vi "Mem_MemoryToLvData_NOPTR.vi"(7 "Type":variant, 8 "error in (no error)":errorcluster, 10 "ByteArray":u8[](array[numeric])) -> (0 "error out":errorcluster, 1 "Supported Type?":bool, 2 "data":variant, 4 "ByteArray Left":u8[](array[numeric]))   [LabVIEW 2019, in "Memory Data Access.lvlib"]
uses:
  Memory Data Access.lvlib
  <vilib>/Utility/Data Type/Type Definitions/Data Type.ctl
  Global/Global.vi
  <vilib>/Utility/Data Type/NI_Data Type.lvlib
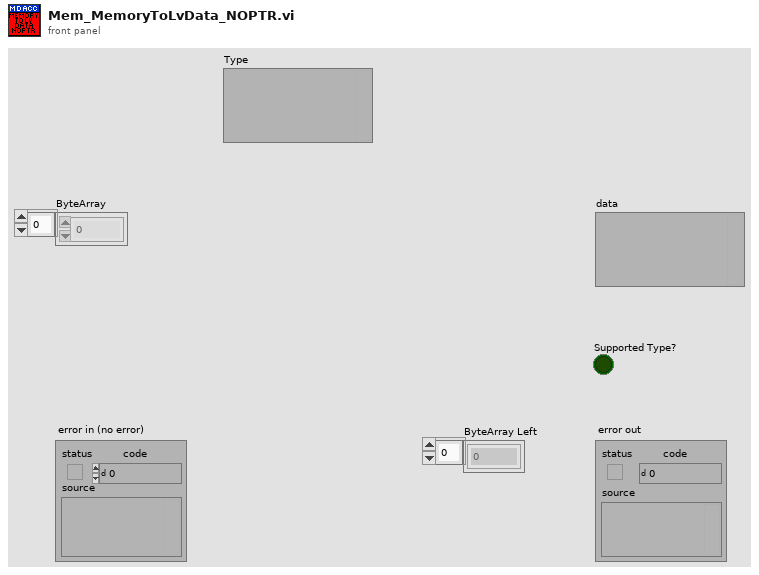
[diagram p1: front panel]
types:
  T1 = typedef "NI_Data Type.lvlib/Data Type.ctl" = enum8{"Invalid Type", "Void", "I8", "I16", "I32", "I64", "U8", "U16", "U32", "U64", "Single Float", "Double Float", "Extended Float", "Single Complex", "Double Complex", "Extended Complex", "Enum U8", "Enum U16", "Enum U32", "Enum U64", "Single Float With Unit", "Double Float With Unit", "Extended Float With Unit", "Single Complex with Unit", "Double Complex with Unit", "Extended Complex with Unit", "Boolean", "String", "Path", "Picture", "Tag", "Array", "Cluster", "Variant", "LV Variant", "Waveform", "Timestamp", "Digital Waveform", "Digital Data", "ExpressData", "Refnum", "External Data", "VI", "Poly VI", "LabVIEW Class Instance", "Fixed Point", "Set Collection", "Map Collection"}
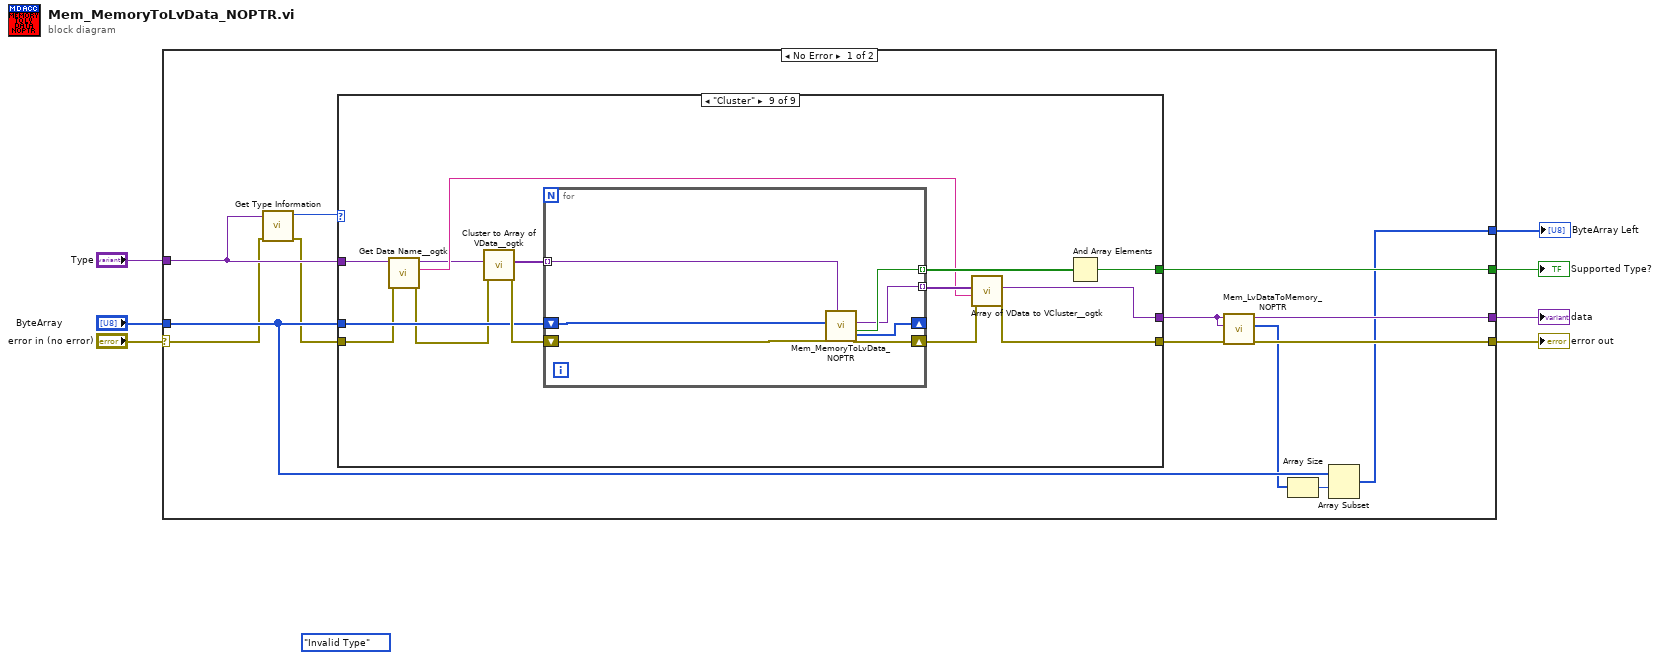
[diagram p0: block diagram]
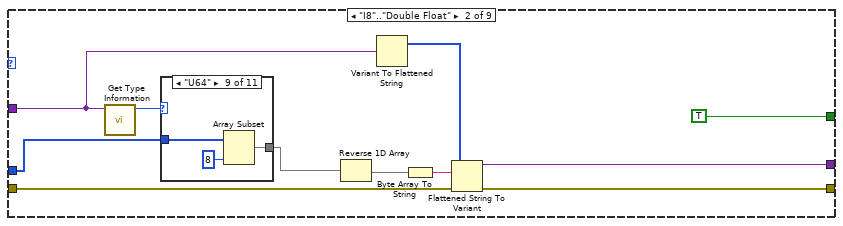
[diagram p3: hidden frame]
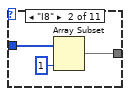
[diagram p5: hidden frame]
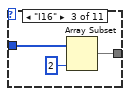
[diagram p6: hidden frame]
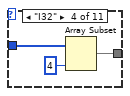
[diagram p7: hidden frame]
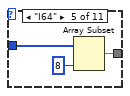
[diagram p8: hidden frame]
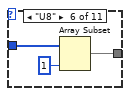
[diagram p9: hidden frame]
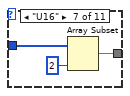
[diagram p10: hidden frame]
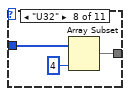
[diagram p11: hidden frame]
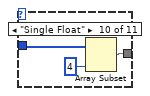
[diagram p12: hidden frame]
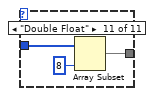
[diagram p13: hidden frame]
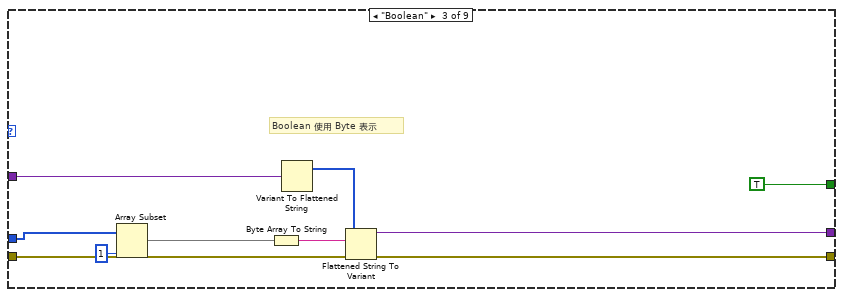
[diagram p14: hidden frame]
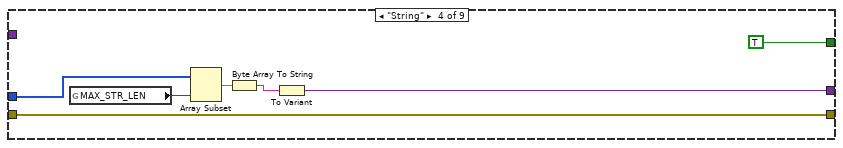
[diagram p15: hidden frame]
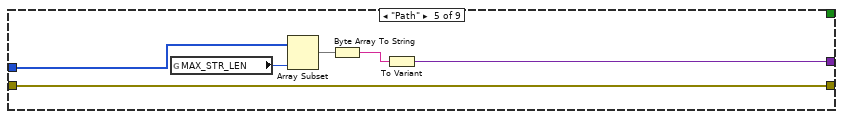
[diagram p16: hidden frame]
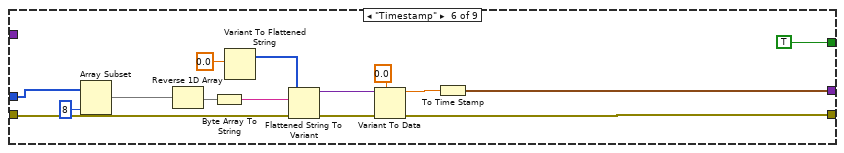
[diagram p17: hidden frame]
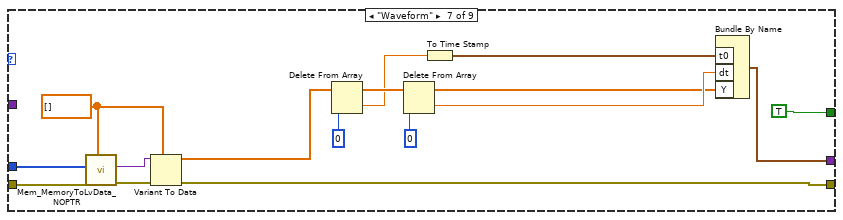
[diagram p18: hidden frame]
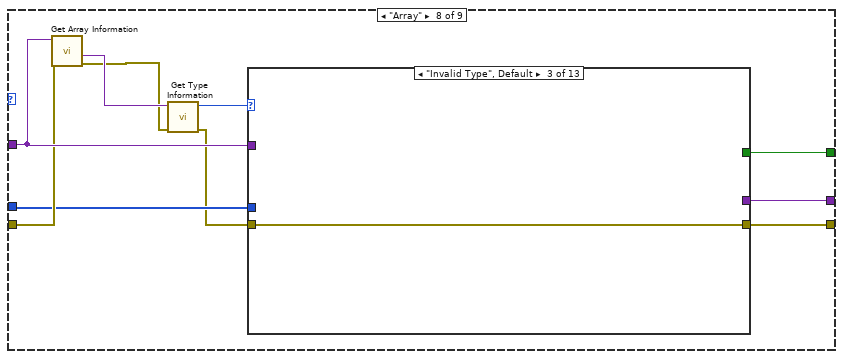
[diagram p19: hidden frame]
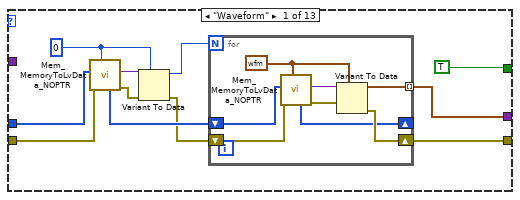
[diagram p20: hidden frame]
diagram:
  (unwired) Data_Type."Invalid Type" ("type")
  n1 = case shown="No Error" "error in (no error)" {
    selector: "error in (no error)" -> [w9 w399]
    tunnel: "ByteArray" -> [w14 _]
    tunnel: [w16 w399] -> w5
    tunnel: "Type" -> [w19 w398]
    tunnel: [w15 w398] -> w3
    tunnel: [w18 _] -> w2
    tunnel: [w13 _] -> w1
    frame No Error {
      n2 = call <vilib>:"Get Type Information.vi"("error in (no error)"=w9, "variant"=w19) -> ("error out"=w8:errorcluster, "type"=w10:T1)  [unwired: 5 in, 3 out]
      n3 = case shown="\"Cluster\"" w10 {
        tunnel: w8 -> [w21 w25 w70 w78 w85 w98 w116 w126 w380]
        tunnel: [w21 w30 w69 w78 w85 w91 w115 w125 w382] -> w17
        tunnel: w19 -> [w20 w22 w72 _ _ _ _ w127 w385]
        tunnel: [_ TRUE TRUE TRUE _ TRUE TRUE w118 w388] -> w18
        tunnel: w14 -> [_ w24 w65 w79 w86 w88 w113 w123 w386]
        tunnel: [w20 w29 w68 w76 w83 w92 w114 w124 w377] -> w15
        frame "Invalid Type", Default {
        }
        frame "I8".."Double Float" {
          n4 = call <vilib>:"Get Type Information.vi"("variant"=w22) -> ("type"=w26:T1)  [unwired: 6 in, 4 out]
          n5 = case shown="\"U64\"" w26 {
            tunnel: w24 -> [w33 w36 w38 w41 w44 w47 w50 w53 w56 w59 w62]
            tunnel: [w33 w34 w37 w40 w43 w46 w49 w52 w55 w58 w61] -> w23
            frame "Invalid Type", Default {
            }
            frame "I8" {
              n6 = Array Subset(array=w36, length=1) -> (w34:u8[])  [unwired: 1 in]
            }
            frame "I16" {
              n7 = Array Subset(array=w38, length=2) -> (w37:u8[])  [unwired: 1 in]
            }
            frame "I32" {
              n8 = Array Subset(array=w41, length=4) -> (w40:u8[])  [unwired: 1 in]
            }
            frame "I64" {
              n9 = Array Subset(array=w44, length=8) -> (w43:u8[])  [unwired: 1 in]
            }
            frame "U8" {
              n10 = Array Subset(array=w47, length=1) -> (w46:u8[])  [unwired: 1 in]
            }
            frame "U16" {
              n11 = Array Subset(array=w50, length=2) -> (w49:u8[])  [unwired: 1 in]
            }
            frame "U32" {
              n12 = Array Subset(array=w53, length=4) -> (w52:u8[])  [unwired: 1 in]
            }
            frame "U64" {
              n13 = Array Subset(array=w56, length=8) -> (w55:u8[])  [unwired: 1 in]
            }
            frame "Single Float" {
              n14 = Array Subset(array=w59, length=4) -> (w58:u8[])  [unwired: 1 in]
            }
            frame "Double Float" {
              n15 = Array Subset(array=w62, length=8) -> (w61:u8[])  [unwired: 1 in]
            }
          }
          n16 = Reverse 1D Array(array=w23) -> (reversed array=w27:u8[])
          n17 = Variant To Flattened String(Variant=w22) -> (1:w31:i16[])  [unwired: 1 out]
          n18 = Byte Array To String(unsigned byte array=w27) -> (string=w28:string)
          n19 = Flattened String To Variant(4:w25, 6:w28, 7:w31) -> (0:w30:errorcluster, 3:w29:variant)
        }
        frame "Boolean" {
          # "Boolean 使用 Byte 表示"
          n20 = Array Subset(array=w65, length=1) -> (w64:u8[])  [unwired: 1 in]
          n21 = Byte Array To String(unsigned byte array=w64) -> (string=w67:string)
          n22 = Variant To Flattened String(Variant=w72) -> (1:w71:i16[])  [unwired: 1 out]
          n23 = Flattened String To Variant(4:w70, 6:w67, 7:w71) -> (0:w69:errorcluster, 3:w68:variant)
        }
        frame "String" {
          n24 = global read "Global.vi" "MAX_STR_LEN"() -> (w74:u32)
          n25 = Array Subset(array=w79, length=w74) -> (w75:u8[])  [unwired: 1 in]
          n26 = Byte Array To String(unsigned byte array=w75) -> (string=w77:string)
          n27 = To Variant(anything=w77) -> (Variant=w76:variant)
        }
        frame "Path" {
          n28 = global read "Global.vi" "MAX_STR_LEN"() -> (w81:u32)
          n29 = Array Subset(array=w86, length=w81) -> (w82:u8[])  [unwired: 1 in]
          n30 = Byte Array To String(unsigned byte array=w82) -> (string=w84:string)
          n31 = To Variant(anything=w84) -> (Variant=w83:variant)
        }
        frame "Timestamp" {
          n32 = Array Subset(array=w88, length=8) -> (w87:u8[])  [unwired: 1 in]
          n33 = Reverse 1D Array(array=w87) -> (reversed array=w99:u8[])
          n34 = Byte Array To String(unsigned byte array=w99) -> (string=w100:string)
          n35 = Variant To Flattened String(Variant=0.0) -> (1:w101:i16[])  [unwired: 1 out]
          n36 = Flattened String To Variant(4:w98, 6:w100, 7:w101) -> (0:w95:errorcluster, 3:w96:variant)
          n37 = Variant To Data(error in=w95, type=0.0, Variant=w96) -> (data=w93:dbl, error out=w91:errorcluster)
          n38 = To Time Stamp(1:w93) -> (0:w92:timestamp)
        }
        frame "Waveform" {
          w102 = dbl[] [] ("array")
          n39 = call "Mem_MemoryToLvData_NOPTR.vi"("Type"=w102, "error in (no error)"=w116, "ByteArray"=w113) -> ("error out"=w104:errorcluster, "data"=w105:variant)  [unwired: 5 in, 2 out]
          n40 = Variant To Data(error in=w104, type=w102, Variant=w105) -> (data=w103:dbl[], error out=w115:errorcluster)
          n41 = Delete From Array(array=w103, index=0) -> (deleted portion=w109:dbl, array with subset deleted=w112:dbl[])  [unwired: 1 in]
          n42 = Delete From Array(array=w112, index=0) -> (deleted portion=w107:dbl, array with subset deleted=w106:dbl[])  [unwired: 1 in]
          n43 = To Time Stamp(1:w109) -> (0:w108:timestamp)
          n44 = Bundle By Name("t0"=w108, "dt"=w107, "Y"=w106) -> (w114:waveform(dbl))  [unwired: 1 in]
        }
        frame "Array" {
          n45 = call <vilib>:"Get Array Information.vi"("error in (no error)"=w126, "variant"=w127) -> ("error out"=w119:errorcluster, "array element data type"=w122:variant)  [unwired: 6 in, 2 out]
          n46 = call <vilib>:"Get Type Information.vi"("error in (no error)"=w119, "variant"=w122) -> ("error out"=w121:errorcluster, "type"=w120:T1)  [unwired: 5 in, 3 out]
          n47 = case shown="\"Invalid Type\", Default" w120 {
            tunnel: w127 -> [_ _ _ _ _ _ _ _ _ _ _ _ _]
            tunnel: w121 -> [w133 w150 w166 w169 w190 w210 w231 w254 w274 w295 w317 w338 w366]
            tunnel: [w130 w148 w166 w169 w190 w210 w231 w254 w274 w295 w317 w338 w366] -> w125
            tunnel: [w129 w149 _ w168 w189 w211 w232 w252 w273 w294 w315 w336 w365] -> w124
            tunnel: w123 -> [w138 w151 _ w170 w191 w212 w233 w253 w275 w296 w316 w337 w364]
            tunnel: [TRUE TRUE _ TRUE TRUE TRUE TRUE TRUE TRUE TRUE TRUE TRUE TRUE] -> w118
            frame "Waveform" {
              w136 = u32 0 ("offset (0)")
              n48 = call "Mem_MemoryToLvData_NOPTR.vi"("Type"=w136, "error in (no error)"=w133, "ByteArray"=w138) -> ("error out"=w135:errorcluster, "data"=w137:variant, "ByteArray Left"=w132:u8[])  [unwired: 5 in, 1 out]
              n49 = Variant To Data(error in=w135, type=w136, Variant=w137) -> (data=w134:u32, error out=w131:errorcluster)
              n50 = for {
                N: w134 -> [_]
                shift-right: [w141] -> w130
                shift-left: w131 -> [w145]
                tunnel: [w142] -> w129 mode=indexing
                shift-right: [w139] -> _
                shift-left: w132 -> [w146]
                w143 = waveform(dbl) {"t0"=timestamp(0 s since 1904-01-01), "dt"=1.0, "Y"=[]} ("Waveform")
                n51 = call "Mem_MemoryToLvData_NOPTR.vi"("Type"=w143, "error in (no error)"=w145, "ByteArray"=w146) -> ("error out"=w140:errorcluster, "data"=w144:variant, "ByteArray Left"=w139:u8[])  [unwired: 5 in, 1 out]
                n52 = Variant To Data(error in=w140, type=w143, Variant=w144) -> (data=w142:waveform(dbl), error out=w141:errorcluster)
              }
            }
            frame "String" {
              w156 = u32 0 ("offset (0)")
              n53 = call "Mem_MemoryToLvData_NOPTR.vi"("Type"=w156, "error in (no error)"=w150, "ByteArray"=w151) -> ("error out"=w155:errorcluster, "data"=w157:variant, "ByteArray Left"=w153:u8[])  [unwired: 5 in, 1 out]
              n54 = Variant To Data(error in=w155, type=w156, Variant=w157) -> (data=w154:u32, error out=w152:errorcluster)
              n55 = for {
                N: w154 -> [_]
                shift-right: [w161] -> w148
                shift-left: w152 -> [w164]
                tunnel: [w162] -> w149 mode=indexing
                shift-right: [w159] -> _
                shift-left: w153 -> [w165]
                w158 = ""
                n56 = call "Mem_MemoryToLvData_NOPTR.vi"("Type"=w158, "error in (no error)"=w164, "ByteArray"=w165) -> ("error out"=w160:errorcluster, "data"=w163:variant, "ByteArray Left"=w159:u8[])  [unwired: 5 in, 1 out]
                n57 = Variant To Data(error in=w160, type=w158, Variant=w163) -> (data=w162:string, error out=w161:errorcluster)
              }
            }
            frame "Invalid Type", Default {
            }
            frame "I8" {
              n58 = Array Subset(array=w170, index=0, length=4) -> (w173:u8[])
              n59 = Reverse 1D Array(array=w173) -> (reversed array=w177:u8[])
              n60 = Type Cast(type=u32 0, x=w177) -> (*(type *) &x=w175:u32)
              n61 = for {
                N: w175 -> [_]
                tunnel: w170 -> [w187]
                tunnel: [w178] -> w176 mode=indexing
                i -> [w186]
                w185 = 1 ("length")
                n62 = Multiply(x=w185, y=w186) -> (x*y=w184:i32)
                n63 = Add(x=4 ("length"), y=w184) -> (x+y=w182:i32)
                n64 = Array Subset(array=w187, index=w182, length=w185) -> (w181:u8[])
                n65 = Reverse 1D Array(array=w181) -> (reversed array=w180:u8[])
                n66 = Type Cast(type=i8 0, x=w180) -> (*(type *) &x=w178:i8)
              }
              n67 = To Variant(anything=w176) -> (Variant=w168:variant)
            }
            frame "I16" {
              n68 = Array Subset(array=w191, index=0, length=4) -> (w194:u8[])
              n69 = Reverse 1D Array(array=w194) -> (reversed array=w198:u8[])
              n70 = Type Cast(type=u32 0, x=w198) -> (*(type *) &x=w196:u32)
              n71 = for {
                N: w196 -> [_]
                tunnel: w191 -> [w208]
                tunnel: [w199] -> w197 mode=indexing
                i -> [w207]
                w206 = 2 ("length")
                n72 = Multiply(x=w206, y=w207) -> (x*y=w205:i32)
                n73 = Add(x=4 ("length"), y=w205) -> (x+y=w203:i32)
                n74 = Array Subset(array=w208, index=w203, length=w206) -> (w202:u8[])
                n75 = Reverse 1D Array(array=w202) -> (reversed array=w201:u8[])
                n76 = Type Cast(type=i16 0, x=w201) -> (*(type *) &x=w199:i16)
              }
              n77 = To Variant(anything=w197) -> (Variant=w189:variant)
            }
            frame "I32" {
              n78 = Array Subset(array=w212, index=0, length=4) -> (w215:u8[])
              n79 = Reverse 1D Array(array=w215) -> (reversed array=w219:u8[])
              n80 = Type Cast(type=u32 0, x=w219) -> (*(type *) &x=w217:u32)
              n81 = for {
                N: w217 -> [_]
                tunnel: w212 -> [w229]
                tunnel: [w220] -> w218 mode=indexing
                i -> [w228]
                w227 = 4 ("length")
                n82 = Multiply(x=w227, y=w228) -> (x*y=w226:i32)
                n83 = Add(x=4 ("length"), y=w226) -> (x+y=w224:i32)
                n84 = Array Subset(array=w229, index=w224, length=w227) -> (w223:u8[])
                n85 = Reverse 1D Array(array=w223) -> (reversed array=w222:u8[])
                n86 = Type Cast(type=0, x=w222) -> (*(type *) &x=w220:i32)
              }
              n87 = To Variant(anything=w218) -> (Variant=w211:variant)
            }
            frame "I64" {
              n88 = Array Subset(array=w233, index=0, length=4) -> (w236:u8[])
              n89 = Reverse 1D Array(array=w236) -> (reversed array=w240:u8[])
              n90 = Type Cast(type=u32 0, x=w240) -> (*(type *) &x=w238:u32)
              n91 = for {
                N: w238 -> [_]
                tunnel: w233 -> [w250]
                tunnel: [w241] -> w239 mode=indexing
                i -> [w249]
                w248 = 8 ("length")
                n92 = Multiply(x=w248, y=w249) -> (x*y=w247:i32)
                n93 = Add(x=4 ("length"), y=w247) -> (x+y=w245:i32)
                n94 = Array Subset(array=w250, index=w245, length=w248) -> (w244:u8[])
                n95 = Reverse 1D Array(array=w244) -> (reversed array=w243:u8[])
                n96 = Type Cast(type=i64 0, x=w243) -> (*(type *) &x=w241:i64)
              }
              n97 = To Variant(anything=w239) -> (Variant=w232:variant)
            }
            frame "U8" {
              n98 = Array Subset(array=w253, index=0, length=4) -> (w257:u8[])
              n99 = Reverse 1D Array(array=w257) -> (reversed array=w261:u8[])
              n100 = Type Cast(type=u32 0, x=w261) -> (*(type *) &x=w259:u32)
              n101 = for {
                N: w259 -> [_]
                tunnel: w253 -> [w271]
                tunnel: [w262] -> w260 mode=indexing
                i -> [w270]
                w269 = 1 ("length")
                n102 = Multiply(x=w269, y=w270) -> (x*y=w268:i32)
                n103 = Add(x=4 ("length"), y=w268) -> (x+y=w266:i32)
                n104 = Array Subset(array=w271, index=w266, length=w269) -> (w265:u8[])
                n105 = Reverse 1D Array(array=w265) -> (reversed array=w264:u8[])
                n106 = Type Cast(type=u8 0, x=w264) -> (*(type *) &x=w262:u8)
              }
              n107 = To Variant(anything=w260) -> (Variant=w252:variant)
            }
            frame "U16" {
              n108 = Array Subset(array=w275, index=0, length=4) -> (w278:u8[])
              n109 = Reverse 1D Array(array=w278) -> (reversed array=w282:u8[])
              n110 = Type Cast(type=u32 0, x=w282) -> (*(type *) &x=w280:u32)
              n111 = for {
                N: w280 -> [_]
                tunnel: w275 -> [w292]
                tunnel: [w283] -> w281 mode=indexing
                i -> [w291]
                w290 = 2 ("length")
                n112 = Multiply(x=w290, y=w291) -> (x*y=w289:i32)
                n113 = Add(x=4 ("length"), y=w289) -> (x+y=w287:i32)
                n114 = Array Subset(array=w292, index=w287, length=w290) -> (w286:u8[])
                n115 = Reverse 1D Array(array=w286) -> (reversed array=w285:u8[])
                n116 = Type Cast(type=u16 0, x=w285) -> (*(type *) &x=w283:u16)
              }
              n117 = To Variant(anything=w281) -> (Variant=w273:variant)
            }
            frame "U32" {
              n118 = Array Subset(array=w296, index=0, length=4) -> (w299:u8[])
              n119 = Reverse 1D Array(array=w299) -> (reversed array=w303:u8[])
              n120 = Type Cast(type=u32 0, x=w303) -> (*(type *) &x=w301:u32)
              n121 = for {
                N: w301 -> [_]
                tunnel: w296 -> [w313]
                tunnel: [w304] -> w302 mode=indexing
                i -> [w312]
                w311 = 4 ("length")
                n122 = Multiply(x=w311, y=w312) -> (x*y=w310:i32)
                n123 = Add(x=4 ("length"), y=w310) -> (x+y=w308:i32)
                n124 = Array Subset(array=w313, index=w308, length=w311) -> (w307:u8[])
                n125 = Reverse 1D Array(array=w307) -> (reversed array=w306:u8[])
                n126 = Type Cast(type=u32 0, x=w306) -> (*(type *) &x=w304:u32)
              }
              n127 = To Variant(anything=w302) -> (Variant=w294:variant)
            }
            frame "U64" {
              n128 = Array Subset(array=w316, index=0, length=4) -> (w320:u8[])
              n129 = Reverse 1D Array(array=w320) -> (reversed array=w324:u8[])
              n130 = Type Cast(type=u32 0, x=w324) -> (*(type *) &x=w322:u32)
              n131 = for {
                N: w322 -> [_]
                tunnel: w316 -> [w334]
                tunnel: [w325] -> w323 mode=indexing
                i -> [w333]
                w332 = 8 ("length")
                n132 = Multiply(x=w332, y=w333) -> (x*y=w331:i32)
                n133 = Add(x=4 ("length"), y=w331) -> (x+y=w329:i32)
                n134 = Array Subset(array=w334, index=w329, length=w332) -> (w328:u8[])
                n135 = Reverse 1D Array(array=w328) -> (reversed array=w327:u8[])
                n136 = Type Cast(type=u64 0, x=w327) -> (*(type *) &x=w325:u64)
              }
              n137 = To Variant(anything=w323) -> (Variant=w315:variant)
            }
            frame "Single Float" {
              n138 = Array Subset(array=w337, index=0, length=4) -> (w341:u8[])
              n139 = Reverse 1D Array(array=w341) -> (reversed array=w345:u8[])
              n140 = Type Cast(type=u32 0, x=w345) -> (*(type *) &x=w343:u32)
              n141 = for {
                N: w343 -> [_]
                tunnel: w337 -> [w355]
                tunnel: [w346] -> w344 mode=indexing
                i -> [w354]
                w353 = 4 ("length")
                n142 = Multiply(x=w353, y=w354) -> (x*y=w352:i32)
                n143 = Add(x=4 ("length"), y=w352) -> (x+y=w350:i32)
                n144 = Array Subset(array=w355, index=w350, length=w353) -> (w349:u8[])
                n145 = Reverse 1D Array(array=w349) -> (reversed array=w348:u8[])
                n146 = Type Cast(type=sgl 0.0, x=w348) -> (*(type *) &x=w346:sgl)
              }
              n147 = To Variant(anything=w344) -> (Variant=w336:variant)
            }
            frame "Double Float" {
              n148 = Array Subset(array=w364, index=0, length=4) -> (w361:u8[])
              n149 = Reverse 1D Array(array=w361) -> (reversed array=w357:u8[])
              n150 = Type Cast(type=u32 0, x=w357) -> (*(type *) &x=w359:u32)
              n151 = for {
                N: w359 -> [_]
                tunnel: w364 -> [w376]
                tunnel: [w367] -> w358 mode=indexing
                i -> [w375]
                w374 = 8 ("length")
                n152 = Multiply(x=w374, y=w375) -> (x*y=w373:i32)
                n153 = Add(x=4 ("length"), y=w373) -> (x+y=w371:i32)
                n154 = Array Subset(array=w376, index=w371, length=w374) -> (w370:u8[])
                n155 = Reverse 1D Array(array=w370) -> (reversed array=w369:u8[])
                n156 = Type Cast(type=0.0, x=w369) -> (*(type *) &x=w367:dbl)
              }
              n157 = To Variant(anything=w358) -> (Variant=w365:variant)
            }
          }
        }
        frame "Cluster" {
          n158 = call <userlib>:"Get Data Name__ogtk.vi"("error in (no error)"=w380, "Data"=w385) -> ("error out"=w381:errorcluster, "Data Name"=w379:string, "Data dup"=w378:variant)  [unwired: 7 in]
          n159 = call <userlib>:"Cluster to Array of VData__ogtk.vi"("error in (no error)"=w381, "Cluster"=w378) -> ("error out"=w387:errorcluster, "Array of VData"=w390:variant[])  [unwired: 8 in]
          n160 = for {
            tunnel: w390 -> [w393] mode=indexing
            tunnel: [w396] -> w389 mode=indexing
            shift-right: [w397] -> w383
            shift-left: w387 -> [w391]
            shift-right: [w394] -> _
            shift-left: w386 -> [w392]
            tunnel: [w395] -> w384 mode=indexing
            n161 = call "Mem_MemoryToLvData_NOPTR.vi"("Type"=w393, "error in (no error)"=w391, "ByteArray"=w392) -> ("error out"=w397:errorcluster, "Supported Type?"=w396:bool, "data"=w395:variant, "ByteArray Left"=w394:u8[])  [unwired: 5 in]
          }
          n162 = call <userlib>:"Array of VData to VCluster__ogtk.vi"("error in (no error)"=w383, "Cluster Name"=w379, "Array"=w384) -> ("error out"=w382:errorcluster, "VCluster"=w377:variant)  [unwired: 7 in]
          n163 = And Array Elements(Boolean array=w389) -> (logical AND=w388:bool)
        }
      }
      n164 = call "Mem_LvDataToMemory_NOPTR.vi"("error in (no error)"=w17, "Payload"=w15) -> ("error out"=w16:errorcluster, "ByteArray"=w12:u8[])  [unwired: 7 in, 1 out]
      n165 = Array Size(array=w12) -> (size(s)=w11:i32)
      n166 = Array Subset(array=w14, index=w11) -> (w13:u8[])  [unwired: 1 in]
    }
    frame Error {
    }
  }
  "error out" <- w5
  "data" <- w3
  "Supported Type?" <- w2
  "ByteArray Left" <- w1
